vi "metadata.update.path.vi"() -> (2 "path":string)   [LabVIEW 2020, in "Nominal Client.lvclass"]
uses:
  Nominal Client/Nominal Client.lvclass
  Nominal Client/Nominal Client.lvclass/Nominal Client.ctl
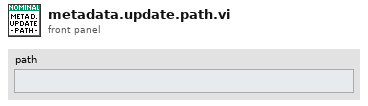
[diagram p1: front panel]
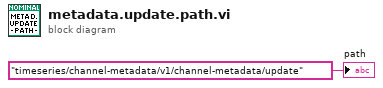
[diagram p0: block diagram]
diagram:
  "path" <- "timeseries/channel-metadata/v1/channel-metadata/update" ("path")
